vi "SendTcpReadyCommand.vi"(6 "機器番号":u8, 9 "TXT In":string, 11 "アドレス":string) -> (1 "送信文字列":string, 2 "空?":bool, 3 "Send List Out":cluster{"Address":string, "Data":string}[](array[cluster]))   [LabVIEW 2017]
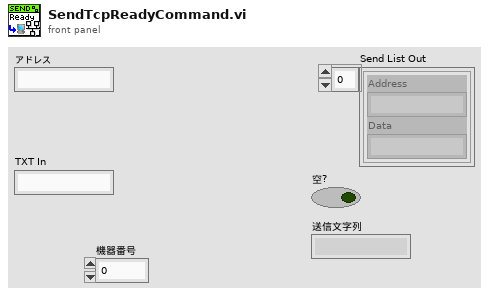
[diagram p1: front panel]
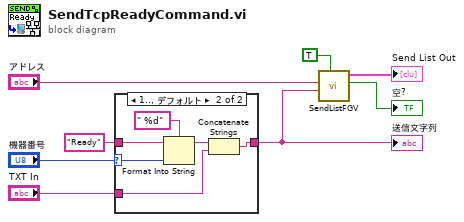
[diagram p0: block diagram]
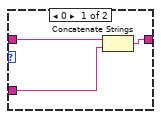
[diagram p2: hidden frame]
diagram:
  n1 = case shown="1.., デフォルト" "機器番号" {
    selector: "機器番号" -> [_ w15]
    tunnel: [w10 w13] -> w8
    tunnel: "Ready" ("要素") -> [w11 w14]
    tunnel: "TXT In" -> [w9 w12]
    frame 0 {
      n2 = Concatenate Strings(w11, w9) -> (w10:string)
    }
    frame 1.., Default {
      n3 = Format Into String(format string=" %d" ("形式文字列"), initial string=w14, w15) -> (resulting string=w17:string)  [unwired: 1 in, 1 out]
      n4 = Concatenate Strings(w17, w12) -> (w13:string)
    }
  }
  "送信文字列" <- w8
  n5 = call "SendListFGV.vi"("Set"=TRUE, "Data"=w8, "アドレス"="アドレス") -> ("空?"=→"空?":bool, "Send List Out"=→"Send List Out":cluster{"Address":string, "Data":string}[])  [unwired: 6 in, 1 out]
